vi "BB_Siren_Run.vi"(6 "Oscillate":bool, 8 "Error In":errorcluster, 9 "sampling info":cluster{"Fs":dbl, "#s":dbl}, 10 "Active":bool, 11 "Task ID In":T1 format="%.0x") -> (0 "error out":errorcluster, 3 "task ID out":T1 format="%.0x")   [LabVIEW 2016]
uses:
  <vilib>/sound2/lvsound2.llb/Sound Output Task ID.ctl
  <vilib>/sound2/lvsound2.llb/Sound Output Set Volume (Single).vi
  <vilib>/sound2/lvsound2.llb/Sound Output Write (DBL Single).vi
  <vilib>/measure/NI_MABase.lvlib
panel:
  in  "High Freq in":dbl=1480.0
  in  "Low Freq in":dbl=440.0
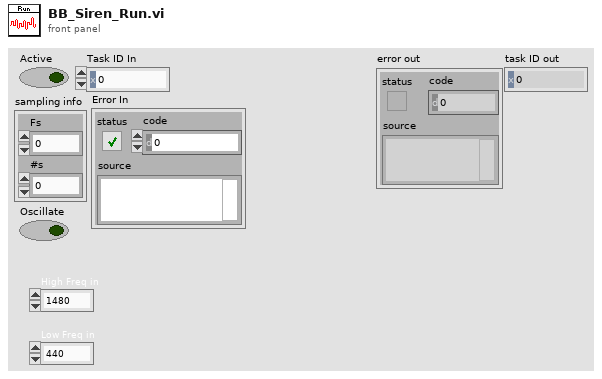
[diagram p1: front panel]
types:
  T1 = typedef "Sound Output Task ID.ctl" = u32
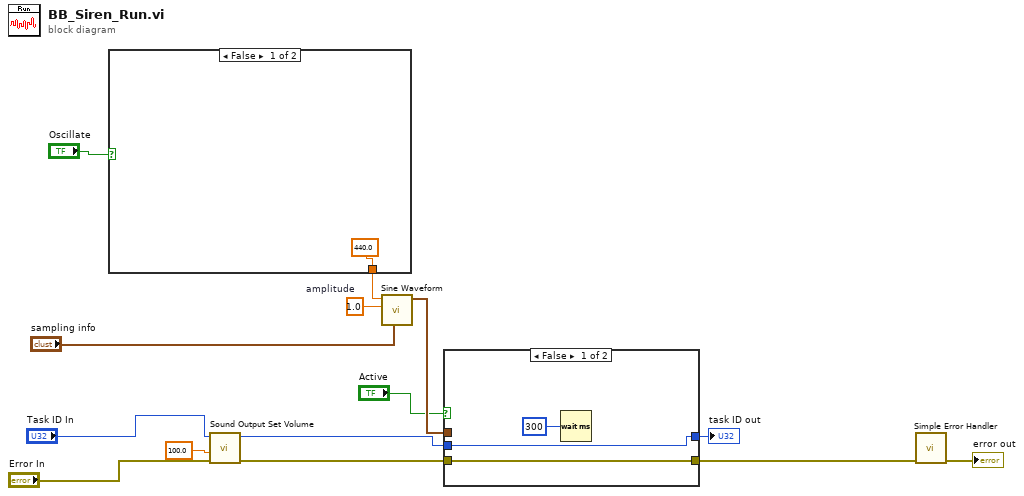
[diagram p0: block diagram]
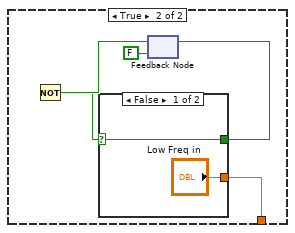
[diagram p2: hidden frame]
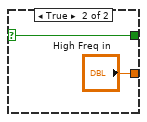
[diagram p3: hidden frame]
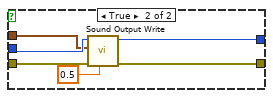
[diagram p4: hidden frame]
diagram:
  w9 = 1.0  # amplitude
  n1 = case shown="False" "Oscillate" {
    tunnel: [440.0 ("High Freq in") w20] -> w10
    frame False {
    }
    frame True {
      n2 = feedback #1(FALSE) -> (w19:bool)
      n3 = Not(x=w19) -> (.not. x?=w16:bool)
      n4 = case shown="False" w16 {
        selector: w16 -> [w21 w23]
        tunnel: ["Low Freq in" "High Freq in"] -> w20
        tunnel: [w21 w23] -> w18
        frame False {
        }
        frame True {
        }
      }
      n5 = feedback-in #1(w18) -> ()
    }
  }
  n6 = call-poly <vilib>:"Sound Output Set Volume.vi"("error in (no error)"="Error In", "volume"=100.0 ("Volume"), "task ID"="Task ID In") -> ("error out"=w8:errorcluster, "task ID out"=w7:T1)  [unwired: 7 in]
  n7 = call <vilib>:"Sine Waveform.vi"("sampling info"="sampling info", "amplitude"=w9, "frequency"=w10) -> ("signal out"=w5:waveform(dbl))  [unwired: 7 in, 1 out]
  n8 = case shown="False" "Active" {
    tunnel: [w26 w33] -> w2
    tunnel: [w25 w32] -> w3
    tunnel: w8 -> [w25 w31]
    tunnel: w7 -> [w26 w30]
    tunnel: w5 -> [_ w29]
    frame False {
      n9 = Wait (ms)(milliseconds to wait=u32 300) -> ()  [unwired: 1 out]
    }
    frame True {
      n10 = call-poly <vilib>:"Sound Output Write.vi"("timeout (sec)"=0.5, "error in (no error)"=w31, "data"=w29, "task ID"=w30) -> ("error out"=w32:errorcluster, "task ID out"=w33:T1)  [unwired: 6 in]
    }
  }
  "task ID out" <- w2
  n11 = call <vilib>:"Simple Error Handler.vi"("error in (no error)"=w3) -> ("error out"=→"error out":errorcluster)  [unwired: 4 in, 4 out]
